vi "Get 1553 Configuration.vi"(8 "error in":errorcluster, 11 "custom device ref":T1 format="%.0x") -> (0 "error out":errorcluster, 2 "1553 configuration out":T2, 3 "custom device ref out":T1 format="%.0x")   [LabVIEW 2020, in "AIM MIL-STD-1553 Engine.lvlib" / "Implementation.lvlib" / "Shared Resources Factory.lvclass"]
uses:
  Shared Resources Factory.lvclass
  Custom Device/Message Configuration.ctl
  Custom Device/Custom Device.lvlib
  Custom Device/Minor Frame Configuration.ctl
  Custom Device/Major Frame Configuration.ctl
  Custom Device/1553 Configuration.ctl
  Scripting/AIM MIL-STD-1553 Scripting.lvlib
  Custom Device/Remote Terminal Configuration.ctl
  Custom Device/Bus Controller Configuration.ctl
  Shared/Direction.ctl
  Custom Device/Acyclic Frame Configuration.ctl
  2f384fe7-c5ea-45c5-b27b-ae7267e18097.vi
  7b96a398-479a-4d68-9f3a-df07bf0e479e.vi
  957f016f-1457-419d-8f79-9cd332dfb9b2.vi
  27c470fe-f49f-4bb1-b96a-3c9ad55f0d32.vi
  <vilib>/NI VeriStand/Custom Device API/Custom Device Item Ref.ctl
  <vilib>/NI VeriStand/Custom Device API/Custom Device API.lvlib
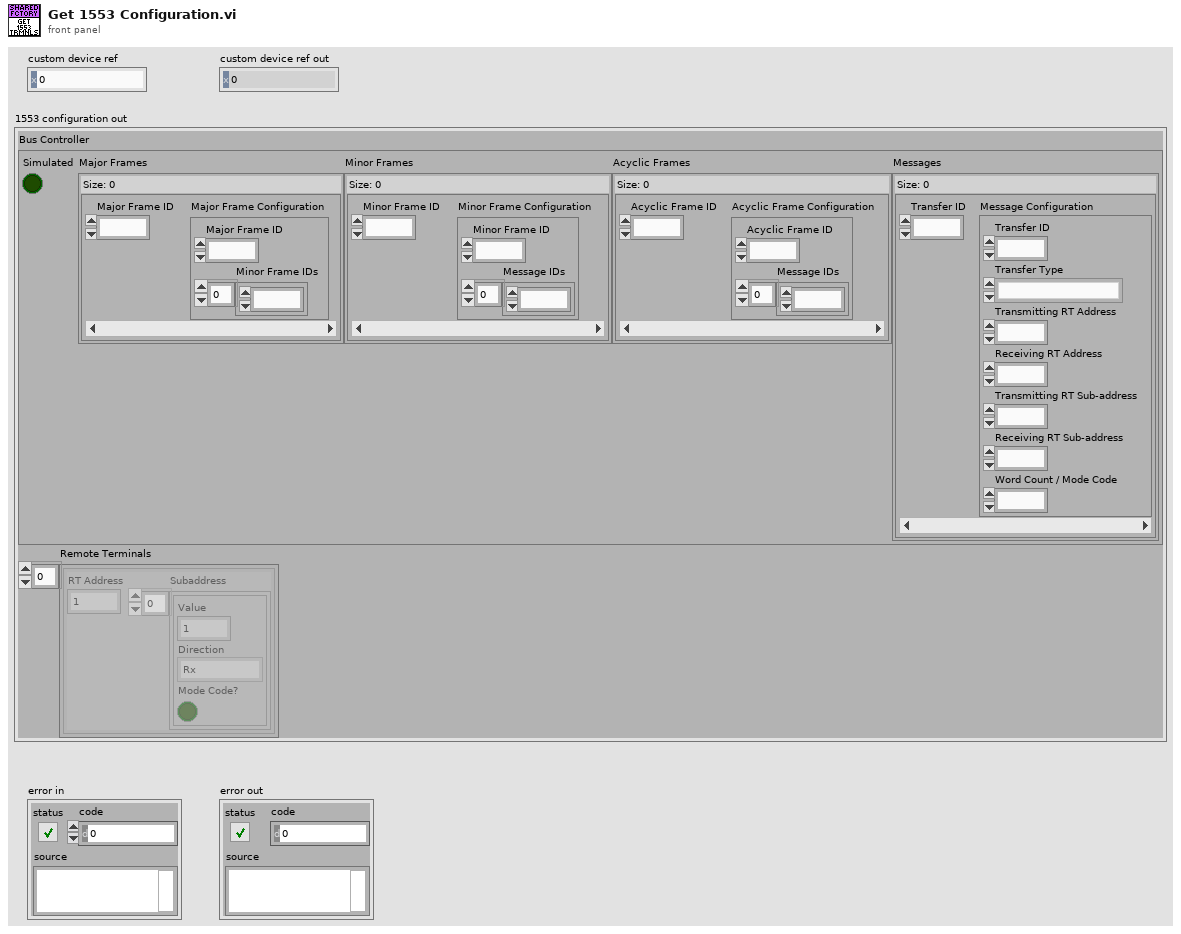
[diagram p1: front panel]
types:
  T1 = typedef "Custom Device API.lvlib/Custom Device Item Ref.ctl" = u64
  T2 = typedef "AIM MIL-STD-1553 Engine.lvlib/Custom Device.lvlib/1553 Configuration.ctl" = cluster{"Bus Controller":T3, "Remote Terminals":T8[]}
  T3 = typedef "AIM MIL-STD-1553 Engine.lvlib/Custom Device.lvlib/Bus Controller Configuration.ctl" = cluster{"Simulated":bool, "Major Frames":map{u8, T4}, "Minor Frames":map{u8, T5}, "Acyclic Frames":map{u8, T6}, "Messages":map{u16, T7}}
  T4 = typedef "AIM MIL-STD-1553 Engine.lvlib/Custom Device.lvlib/Major Frame Configuration.ctl" = cluster{"Major Frame ID":u8, "Minor Frame IDs":u8[]}
  T5 = typedef "AIM MIL-STD-1553 Engine.lvlib/Custom Device.lvlib/Minor Frame Configuration.ctl" = cluster{"Minor Frame ID":u8, "Message IDs":u16[]}
  T6 = typedef "AIM MIL-STD-1553 Engine.lvlib/Custom Device.lvlib/Acyclic Frame Configuration.ctl" = cluster{"Acyclic Frame ID":u8, "Message IDs":u16[]}
  T7 = typedef "AIM MIL-STD-1553 Engine.lvlib/Custom Device.lvlib/Message Configuration.ctl" = cluster{"Transfer ID":u16, "Transfer Type":enum16{"BC to RT transfer", "RT to BC transfer", "RT to RT transfer"}, "Transmitting RT Address":u8, "Receiving RT Address":u8, "Transmitting RT Sub-address":u8, "Receiving RT Sub-address":u8, "Word Count / Mode Code":u8}
  T8 = typedef "AIM MIL-STD-1553 Engine.lvlib/Custom Device.lvlib/Remote Terminal Configuration.ctl" = cluster{"RT Address":u8, "Subaddress":cluster{"Value":u8, "Direction":T9, "Mode Code?":bool}[]}
  T9 = typedef "Direction.ctl" = enum16{"Rx", "Tx"}
  T10 = typedef "Acyclic Frame Definition.ctl" = cluster{"name":string, "messages":string[]}
  T11 = typedef "Message Definition.ctl" = cluster{"name":string, "message type":T12, "endpoint Tx":T13, "endpoint Rx":T13, "create timestamp channel":bool, "mode code":u16, "number of words":u16, "parameters":cluster{"name":string, "default value":dbl, "unit":string, "parameter definition":T15}[]}
  T12 = typedef "Message Type.ctl" = string
  T13 = typedef "Terminal Endpoint.ctl" = cluster{"terminal address":T14, "subaddress":T14}
  T14 = typedef "Address.ctl" = u16
  T15 = typedef "Parameter Definition.ctl" = cluster{"start index":i32, "size (bits)":i32, "encoding":enum16{"BNR", "BCD", "Discrete"}, "signed":bool, "multiplier":dbl, "offset":dbl}
  T16 = typedef "Minor Frame Definition.ctl" = cluster{"name":string, "messages":string[]}
  T17 = typedef "Major Frame Definition.ctl" = cluster{"name":string, "minor frames":string[]}
  T18 = cluster{"Value":u8, "Direction":T9, "Mode Code?":bool}
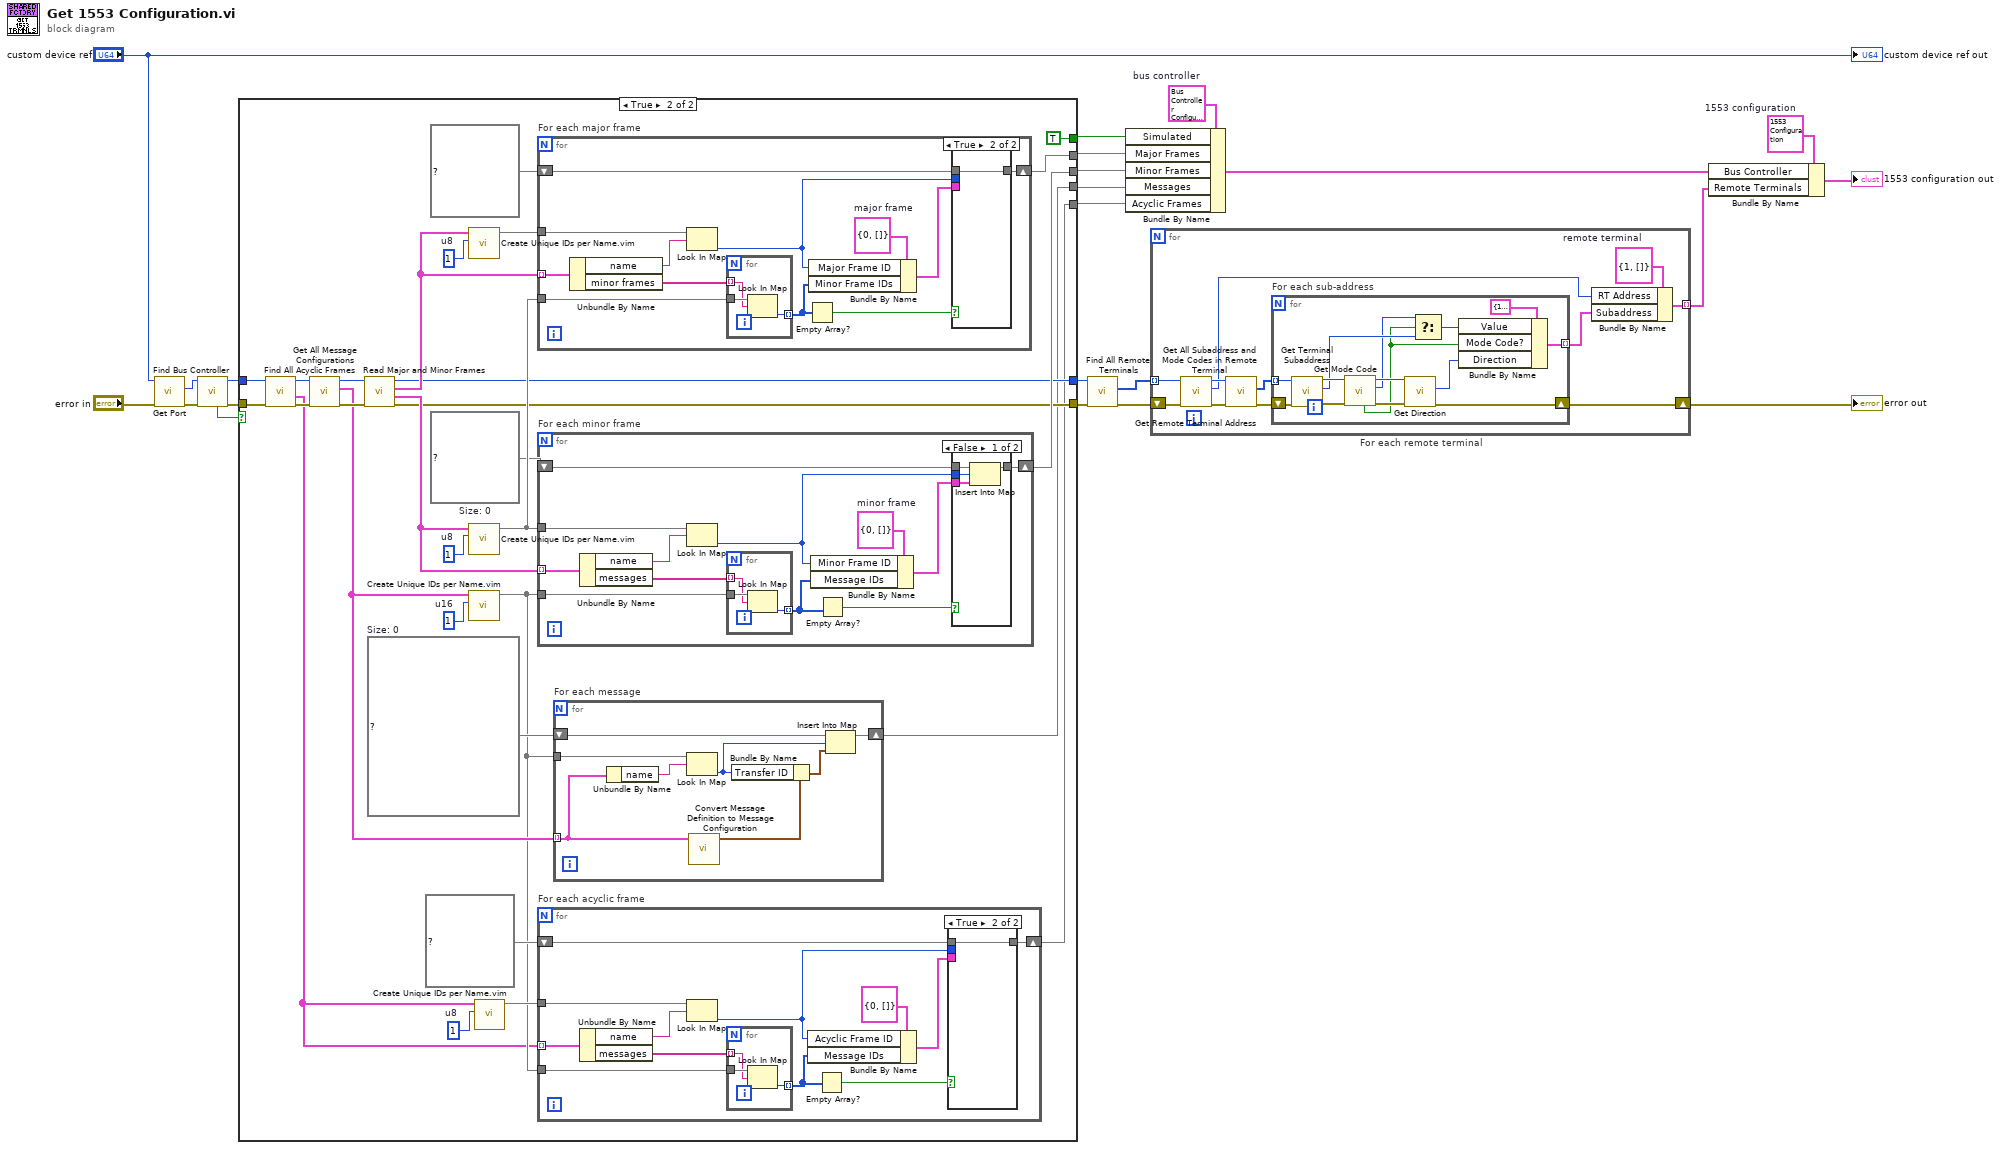
[diagram p0: block diagram]
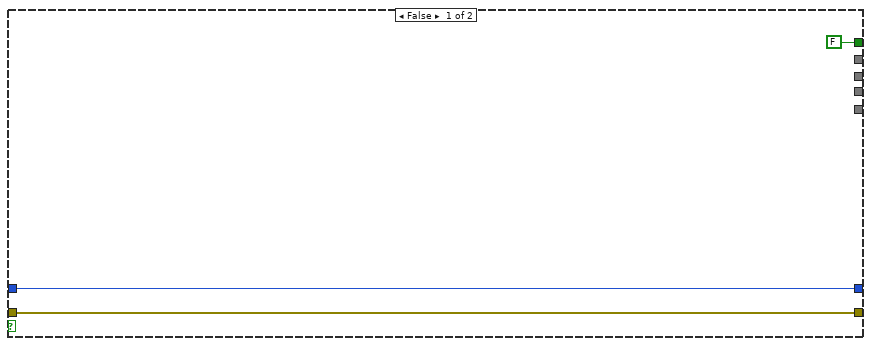
[diagram p2: hidden frame]
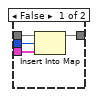
[diagram p3: hidden frame]
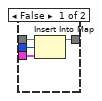
[diagram p5: hidden frame]
diagram:
  w21 = T3 {"Simulated"=FALSE, "Major Frames"={}, "Minor Frames"={}, "Acyclic Frames"={}, "Messages"={}}  # bus controller
  w22 = T2 {"Bus Controller"={"Simulated"=FALSE, "Major Frames"={}, "Minor Frames"={}, "Acyclic Frames"={}, "Messages"={}}, "Remote Terminals"=[]}  # 1553 configuration
  n1 = call "Get Port.vi"("error in"="error in", "custom device ref"="custom device ref") -> ("error out"=w5:errorcluster, "port"=w3:T1)  [unwired: 6 in, 2 out]
  n2 = call "Find Bus Controller.vi"("error in"=w5, "port"=w3) -> ("error out"=w18:errorcluster, "port out"=w17:T1, "found?"=w16:bool)  [unwired: 6 in, 1 out]
  n3 = case shown="True" w16 {
    tunnel: [_ w46] -> w20
    tunnel: [_ w45] -> w19
    tunnel: w18 -> [w24 w30]
    tunnel: w17 -> [w23 w28]
    tunnel: [FALSE TRUE] -> w15
    tunnel: [_ w36] -> w1
    tunnel: [w24 w39] -> w11
    tunnel: [w23 w38] -> w12
    tunnel: [_ w37] -> w2
    frame False {
    }
    frame True {
      w33 = u8 1  # u8
      w40 = map{u16, T7} {}  # Size: 0
      w41 = map{u8, T5} {}  # Size: 0
      w50 = u16 1  # u16
      w51 = u8 1  # u8
      w52 = u8 1  # u8
      n4 = call "Find All Acyclic Frames.vi"("error in"=w30, "port"=w28) -> ("error out"=w29:errorcluster, "acyclic frames"=w26:T10[], "port out"=w27:T1)  [unwired: 6 in, 1 out]
      n5 = call "Get All Message Configurations.vi"("error in"=w29, "port"=w27) -> ("error out"=w44:errorcluster, "message configurations"=w34:T11[], "port out"=w43:T1)  [unwired: 7 in]
      n6 = call "Read Major and Minor Frames.vi"("error in"=w44, "port"=w43) -> ("error out"=w39:errorcluster, "minor frames"=w47:T16[], "major frames"=w54:T17[], "port out"=w38:T1)  [unwired: 6 in]
      n7 = call "Create Unique IDs per Name.vim"("starting id value"=w51, "array"=w54) -> ("names to ids"=w53:map{string, u8})  [unwired: 9 in]
      n8 = call "Create Unique IDs per Name.vim"("starting id value"=w52, "array"=w47) -> ("names to ids"=w48:map{string, u8})  [unwired: 9 in]
      n9 = call "Create Unique IDs per Name.vim"("starting id value"=w50, "array"=w34) -> ("names to ids"=w31:map{string, u16})  [unwired: 9 in]
      n10 = call "Create Unique IDs per Name.vim"("starting id value"=w33, "array"=w26) -> ("names to ids"=w32:map{string, u8})  [unwired: 9 in]
      n11 = for "For each major frame" {
        tunnel: w54 -> [w114] mode=indexing
        tunnel: w53 -> [w113]
        tunnel: w48 -> [w110]
        shift-right: [w107] -> w46
        shift-left: map{u8, T4} {} ("Major Frames") -> [w108]
        w109 = T4 {"Major Frame ID"=0, "Minor Frame IDs"=[]}  # major frame
        n12 = Unbundle By Name(w114) -> ("name"=w112:string, "minor frames"=w111:string[])
        n13 = Look In Map(map=w113, key=w112) -> (value=w105:u8)  [unwired: 1 in, 1 out]
        n14 = for {
          tunnel: w111 -> [w121] mode=indexing
          tunnel: w110 -> [w122]
          tunnel: [w120] -> w104 mode=indexing
          n15 = Look In Map(map=w122, key=w121) -> (value=w120:u8)  [unwired: 1 in, 1 out]
        }
        n16 = Empty Array?(array=w104) -> (empty?=w103:bool)
        n17 = Bundle By Name(cluster=w109, "Major Frame ID"=w105, "Minor Frame IDs"=w104) -> (w106:T4)
        n18 = case shown="True" w103 {
          tunnel: w108 -> [w118 w119]
          tunnel: [w117 w119] -> w107
          tunnel: w106 -> [w116 _]
          tunnel: w105 -> [w115 _]
          frame False {
            n19 = Insert Into Map(map in=w118, key=w115, value=w116) -> (map out=w117:map{u8, T4})  [unwired: 2 out]
          }
          frame True {
          }
        }
      }
      n20 = for "For each minor frame" {
        tunnel: w47 -> [w94] mode=indexing
        tunnel: w48 -> [w93]
        tunnel: w31 -> [w90]
        shift-right: [w87] -> w45
        shift-left: w41 -> [w88]
        w89 = T5 {"Minor Frame ID"=0, "Message IDs"=[]}  # minor frame
        n21 = Unbundle By Name(w94) -> ("name"=w92:string, "messages"=w91:string[])
        n22 = Look In Map(map=w93, key=w92) -> (value=w85:u8)  [unwired: 1 in, 1 out]
        n23 = for {
          tunnel: w91 -> [w101] mode=indexing
          tunnel: w90 -> [w102]
          tunnel: [w100] -> w84 mode=indexing
          n24 = Look In Map(map=w102, key=w101) -> (value=w100:u16)  [unwired: 1 in, 1 out]
        }
        n25 = Bundle By Name(cluster=w89, "Minor Frame ID"=w85, "Message IDs"=w84) -> (w86:T5)
        n26 = Empty Array?(array=w84) -> (empty?=w83:bool)
        n27 = case shown="False" w83 {
          tunnel: w88 -> [w98 w99]
          tunnel: [w97 w99] -> w87
          tunnel: w86 -> [w96 _]
          tunnel: w85 -> [w95 _]
          frame False {
            n28 = Insert Into Map(map in=w98, key=w95, value=w96) -> (map out=w97:map{u8, T5})  [unwired: 2 out]
          }
          frame True {
          }
        }
      }
      n29 = for "For each acyclic frame" {
        tunnel: w26 -> [w66] mode=indexing
        tunnel: w32 -> [w65]
        tunnel: w31 -> [w62]
        shift-right: [w60] -> w36
        shift-left: map{u8, T6} {} ("Acyclic Frames") -> [w61]
        n30 = Unbundle By Name(w66) -> ("name"=w64:string, "messages"=w63:string[])
        n31 = Look In Map(map=w65, key=w64) -> (value=w58:u8)  [unwired: 1 in, 1 out]
        n32 = for {
          tunnel: w63 -> [w73] mode=indexing
          tunnel: w62 -> [w74]
          tunnel: [w72] -> w55 mode=indexing
          n33 = Look In Map(map=w74, key=w73) -> (value=w72:u16)  [unwired: 1 in, 1 out]
        }
        n34 = Bundle By Name(cluster=T6 {"Acyclic Frame ID"=0, "Message IDs"=[]} ("Acyclic Frame Configuration"), "Acyclic Frame ID"=w58, "Message IDs"=w55) -> (w59:T6)
        n35 = Empty Array?(array=w55) -> (empty?=w56:bool)
        n36 = case shown="True" w56 {
          tunnel: w61 -> [w70 w71]
          tunnel: [w69 w71] -> w60
          tunnel: w59 -> [w68 _]
          tunnel: w58 -> [w67 _]
          frame False {
            n37 = Insert Into Map(map in=w70, key=w67, value=w68) -> (map out=w69:map{u8, T6})  [unwired: 2 out]
          }
          frame True {
          }
        }
      }
      n38 = for "For each message" {
        tunnel: w34 -> [w76] mode=indexing
        tunnel: w31 -> [w82]
        shift-right: [w79] -> w37
        shift-left: w40 -> [w80]
        n39 = Unbundle By Name(w76) -> ("name"=w81:string)
        n40 = Look In Map(map=w82, key=w81) -> (value=w77:u16)  [unwired: 1 in, 1 out]
        n41 = call "Convert Message Definition to Message Configuration.vi"("message definition"=w76) -> ("message configuration"=w75:T7)  [unwired: 10 in]
        n42 = Bundle By Name(cluster=w75, "Transfer ID"=w77) -> (w78:T7)
        n43 = Insert Into Map(map in=w80, key=w77, value=w78) -> (map out=w79:map{u16, T7})  [unwired: 2 out]
      }
    }
  }
  n44 = call "Find All Remote Terminals.vi"("error in"=w11, "port"=w12) -> ("error out"=w9:errorcluster, "remote terminals"=w10:T1[])  [unwired: 7 in, 1 out]
  n45 = Bundle By Name(cluster=w21, "Simulated"=w15, "Major Frames"=w20, "Minor Frames"=w19, "Messages"=w2, "Acyclic Frames"=w1) -> (w14:T3)
  n46 = for "For each remote terminal" {
    tunnel: w10 -> [w132] mode=indexing
    shift-right: [w131] -> w7
    shift-left: w9 -> [w133]
    tunnel: [w123] -> w8 mode=indexing
    w126 = T8 {"RT Address"=1, "Subaddress"=[]}  # remote terminal
    n47 = call "Get Remote Terminal Address.vi"("error in"=w133, "remote terminal"=w132) -> ("error out"=w129:errorcluster, "terminal address"=w125:T14, "remote terminal out"=w130:T1)  [unwired: 6 in, 1 out]
    n48 = call "Get All Subaddress and Mode Codes in Remote Terminal.vi"("error in"=w129, "remote terminal"=w130) -> ("error out"=w128:errorcluster, "subaddress sections"=w127:T1[])  [unwired: 7 in, 1 out]
    n49 = for "For each sub-address" {
      shift-right: [w145] -> w131
      shift-left: w128 -> [w147]
      tunnel: w127 -> [w146] mode=indexing
      tunnel: [w144] -> w124 mode=indexing
      n50 = call "Get Terminal Subaddress.vi"("error in"=w147, "subaddress section"=w146) -> ("error out"=w142:errorcluster, "subaddress value"=w137:T14, "subaddress section out"=w143:T1)  [unwired: 6 in, 1 out]
      n51 = call "Get Mode Code.vi"("error in"=w142, "message or subaddress"=w143) -> ("error out"=w141:errorcluster, "mode code"=w136:u16, "message or subaddress out"=w140:T1, "found?"=w135:bool)  [unwired: 6 in]
      n52 = call "Get Direction.vi"("error in"=w141, "message or subaddress"=w140) -> ("error out"=w145:errorcluster, "direction"=w139:T9)  [unwired: 6 in, 2 out]
      n53 = Select(t=w136, s=w135, f=w137) -> (s? t:f=w138:T14)
      n54 = Bundle By Name(cluster=T18 {"Value"=1, "Direction"=enum."Rx", "Mode Code?"=FALSE} ("Subaddress"), "Value"=w138, "Mode Code?"=w135, "Direction"=w139) -> (w144:T18)
    }
    n55 = Bundle By Name(cluster=w126, "RT Address"=w125, "Subaddress"=w124) -> (w123:T8)
  }
  "error out" <- w7
  n56 = Bundle By Name(cluster=w22, "Bus Controller"=w14, "Remote Terminals"=w8) -> (→"1553 configuration out":T2)
  "custom device ref out" <- "custom device ref"
